vi "ROI entry-Exit actions.vi"(9 "Imaging Mode":T2, 10 "Stop loop":bool, 11 "User Events cluster":T1) -> (0 "error out":errorcluster)   [LabVIEW 2020]
uses:
  Typedefs/Top level VI states.ctl
  Typedefs/Offsets cluster.ctl
  Typedefs/Imaging Protocols enum.ctl
  Global Variables/gl_Queues.vi
  Global Variables/General Globals.vi
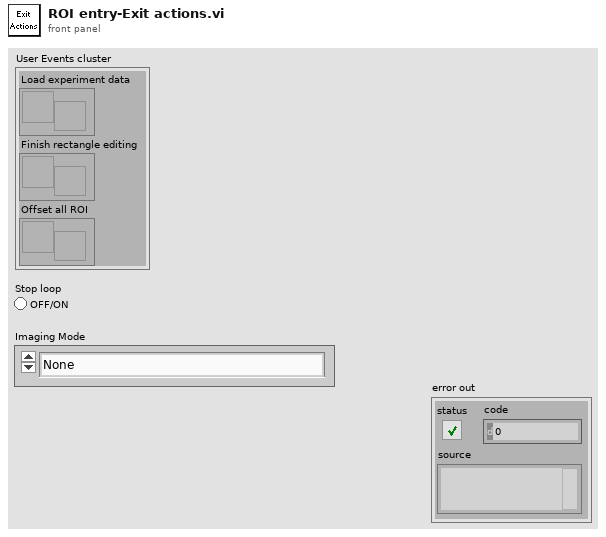
[diagram p1: front panel]
types:
  T1 = cluster{"Load experiment data":refnum<user-event>, "Finish rectangle editing":refnum<user-event>, "Offset all ROI":refnum<user-event>}
  T2 = typedef "Top level VI states.ctl" = enum16{"None", "Initialise UI", "<STACK PROTOCOL STATES>", "AOL Zstack-START", "AOL Zstack-STOP", "Motor Zstack-START", "Motor Zstack-STOP", "<ACQUISITION PROTOCOL STATES> ", "Functional Acquisition-START", "Functional Acquisition-STOP", "Single Plane Acquisition-START", "Single Plane Acquisition-STOP", "Volume Acquisition-START", "Volume Acquisition-STOP", "<LIVE IMAGING PROTOCOL STATES>", "Live Imaging-START", "Live Imaging-STOP", "Live Plane Imaging-START", "Live Plane Imaging-STOP", "Live Volume Imaging-START", "Live Volume Imaging-STOP", "<MOVEMENT CORRECTION PROTOCOL STATES>", "EXIT"}
  T3 = typedef "Imaging Protocols enum.ctl" = enum16{"AOL Z-Stack", "Motor Z Stack", "Functional Acquisition", "Single Plane Acquisition", "Volume Acquisition", "Live Imaging", "Live Plane Imaging", "Live Volume Imaging"}
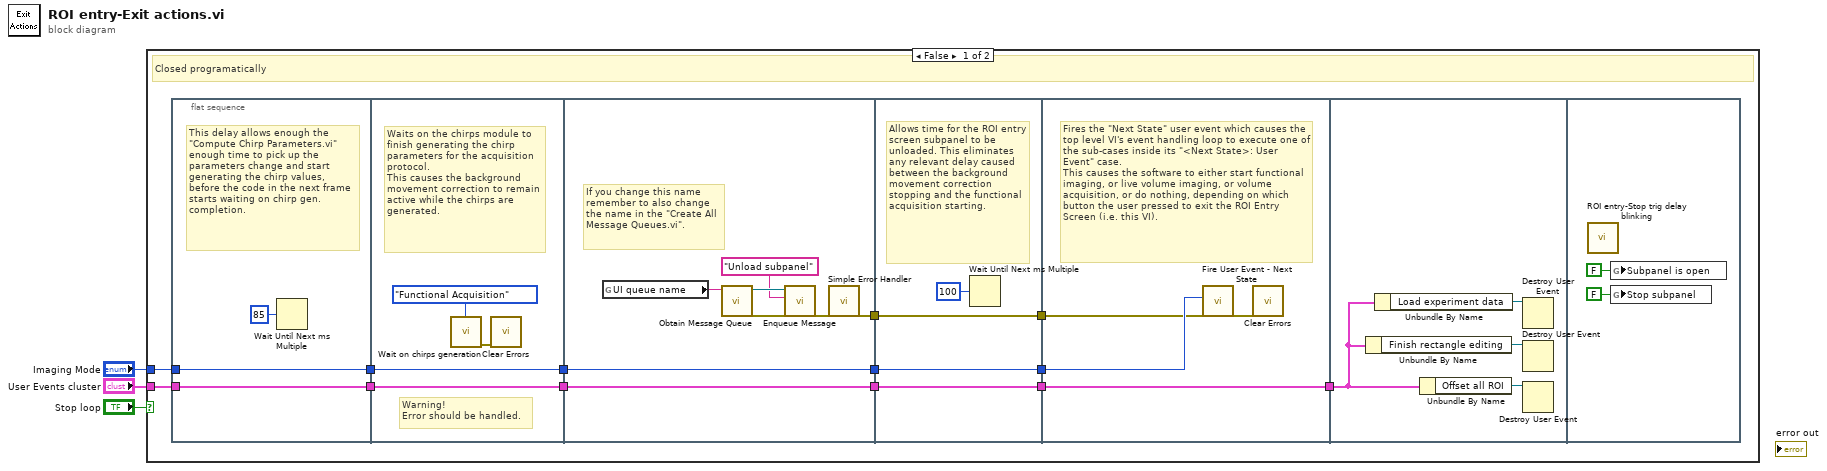
[diagram p0: block diagram]
diagram:
  n1 = case shown="False" "Stop loop" {
    tunnel: "User Events cluster" -> [w14 _]
    tunnel: "Imaging Mode" -> [w16 _]
    frame False {
      # "Closed programatically"
      n2 = flat-sequence {
        tunnel: [w19] -> w13
        tunnel: [w18] -> w12
        tunnel: w16 -> [w19]
        tunnel: w14 -> [w18]
        tunnel: w13 -> [w23]
        tunnel: [w23] -> w11
        tunnel: w12 -> [w22]
        tunnel: [w22] -> w10
        tunnel: w11 -> [w31]
        tunnel: [w31] -> w9
        tunnel: w10 -> [w30]
        tunnel: [w30] -> w7
        tunnel: [w25] -> w5
        tunnel: w9 -> [w35]
        tunnel: [w35] -> w8
        tunnel: w7 -> [w34]
        tunnel: [w34] -> w6
        tunnel: w5 -> [w33]
        tunnel: [w33] -> w4
        tunnel: w8 -> [w39]
        tunnel: [w37] -> w15
        tunnel: w6 -> [w37]
        tunnel: w4 -> [w36]
        tunnel: w15 -> [w40]
        frame #0 {
          # "This delay allows enough the \"Compute Chirp Parameters.vi\" enough time to pick up the parameters change and start generating the chirp values, before the code in the next frame starts waiting on chirp gen. completion."
          n3 = Wait Until Next ms Multiple(millisecond multiple=u32 85) -> ()  [unwired: 1 out]
        }
        frame #1 {
          # "Warning!\nError should be handled."
          # "Waits on the chirps module to finish generating the chirp parameters for the acquisition protocol.\nThis causes the background movement correction to remain active while the chirps are generated."
          n4 = call "Wait on chirps generation.vi"("Imaging Protocol"=Imaging_Protocols_enum."Functional Acquisition") -> ("error out"=w20:errorcluster)  [unwired: 9 in, 1 out]
          n5 = call <vilib>:"Clear Errors.vi"("error in (no error)"=w20) -> ()  [unwired: 5 in, 2 out]
        }
        frame #2 {
          # "If you change this name remember to also change the name in the \"Create All Message Queues.vi\"."
          n6 = global read "gl_Queues.vi" "UI queue name"() -> (w24:string)
          n7 = call "Obtain Message Queue.vi"("Queue name"=w24) -> ("error out"=w29:errorcluster, "Message Queue"=w28:refnum<queue>)  [unwired: 9 in]
          n8 = call "Enqueue Message.vi"("error in (no error)"=w29, "Message"="Unload subpanel", "Queue"=w28) -> ("error out"=w26:errorcluster)  [unwired: 7 in, 1 out]
          n9 = call <vilib>:"Simple Error Handler.vi"("error in (no error)"=w26) -> ("error out"=w25:errorcluster)  [unwired: 4 in, 4 out]
        }
        frame #3 {
          # "Allows time for the ROI entry screen subpanel to be unloaded. This eliminates any relevant delay caused between the background movement correction stopping and the functional acquisition starting."
          n10 = Wait Until Next ms Multiple(millisecond multiple=u32 100) -> ()  [unwired: 1 out]
        }
        frame #4 {
          # "Fires the \"Next State\" user event which causes the top level VI's event handling loop to execute one of the sub-cases inside its \"<Next State>: User Event\" case.\nThis causes the software to either start functional imaging, or live volume imaging, or volume acquisition, or do nothing, depending on which button the user pressed to exit the ROI Entry Screen (i.e. this VI)."
          n11 = call "Fire User Event - Next State.vi"("Error In"=w36, "\"UI Handler loop\" case to execute"=w39) -> ("Error Out"=w38:errorcluster)  [unwired: 9 in]
          n12 = call <vilib>:"Clear Errors.vi"("error in (no error)"=w38) -> ()  [unwired: 5 in, 2 out]
        }
        frame #5 {
          n13 = Unbundle By Name(w40) -> ("Finish rectangle editing"=w42:refnum<user-event>)
          n14 = Unbundle By Name(w40) -> ("Load experiment data"=w43:refnum<user-event>)
          n15 = Unbundle By Name(w40) -> ("Offset all ROI"=w41:refnum<user-event>)
          n16 = Destroy User Event(user event=w43) -> ()  [unwired: 1 in, 1 out]
          n17 = Destroy User Event(user event=w42) -> ()  [unwired: 1 in, 1 out]
          n18 = Destroy User Event(user event=w41) -> ()  [unwired: 1 in, 1 out]
        }
        frame #6 {
          n19 = call "ROI entry-Stop trig delay blinking.vi"() -> ()  [unwired: 12 in]
          n20 = global write "General Globals.vi" "Subpanel is open"(FALSE ("Subpanel is open")) -> ()
          n21 = global write "General Globals.vi" "Stop subpanel"(FALSE ("Stop subpanel")) -> ()
        }
      }
    }
    frame True {
      # "Window closed manually during development."
    }
  }
